vi "Set Status To String.vi"(2 "Status type":refnum<class "Status.lvclass">, 3 "Status":variant, 4 "Item Name":string, 5 "Sender":string) -> (1 "data string":string)   [LabVIEW 2017, in "Message Interface.lvlib" / "Status.lvclass"]
uses:
  Status.lvclass
  Volumes/Data/Users/benji667/Git/BuildFarm/BuildWorker/Classes/iMessage/iMessage.lvclass
  iMessage/iMessage.lvclass/iMessage.ctl
  Status.lvclass/Status.ctl
  iMessage/Write Sender.vi
  Write Item Name.vi
  Write Status.vi
  iMessage/iMessage.lvclass
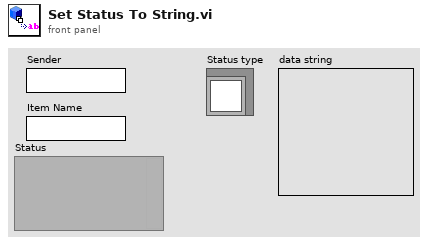
[diagram p1: front panel]
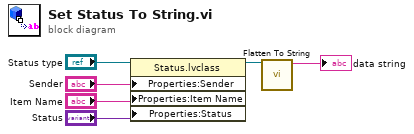
[diagram p0: block diagram]
diagram:
  n1 = property class="Status.lvclass"(reference="Status type", "Properties:Sender"="Sender", "Properties:Item Name"="Item Name", "Properties:Status"="Status") -> (reference out=w2:refnum<class "Status.lvclass">)  [unwired: 1 in, 1 out]
  n2 = call "Flatten To String.vi"("iMessage in"=w2) -> ("data string"=→"data string":string)  [unwired: 9 in, 1 out]
